vi "Error.Format.vi"(5 "[user-defined descriptions]":string[](array[string]), 7 "[user-defined codes]":i32[](array[numeric]), 8 "error in (no error)":errorcluster, 10 "[error source] (\" \")":string, 11 "[error code] (0)":i32 format="%0.0f") -> (0 "error out":errorcluster, 1 "source out":string, 2 "code out":i32 format="%0.0f", 3 "error?":bool, 4 "message":string=" INSTRUCTIONS:\r\rNormal Use:  When using subVIs that incorporate the error in/error out (or error I/O) structure, place this handler where you want to inform the user of an error, typically at the end of the I/O data path, as the last action of the program.  If the error in error? is ERROR, the handler creates a message describing the error and its source.  If the type of dialog = 1 (default), the message is displayed to the user, who can only acknowedge it.  If the type = 2, the user can acknowledge the message or abort execution; aborting a program with active I/O is not recommended.  If the type = 0, no message is displayed; this is used to process the error programmatically, and the error out cluster elements are wired to individual terminals for that reason.  \r\rOther Use:\n\r\nlocal testing.  To test the error code of a subVI or function that does not have the error I/O structure, you can wire its error code and a source string to the local error code and error source inputs.  If error in error? indicates no error and error code is not equal to 0, the local code and source are substituted for the error in values, and error? is set TRUE (ERROR).")   [LabVIEW 2023, in "VS Plugin Inline Async API.lvlib"]
uses:
  VS Plugin Inline Async API.lvlib
  <vilib>/Utility/error.llb/whitespace.ctl
  <vilib>/Utility/error.llb/Trim Whitespace One-Sided.vi
  <vilib>/Utility/error.llb/Find Tag.vi
panel:
  in  "prompts":T1={"Error %d occurred at %s"="Error %d occurred at %s", "Warning %d occurred at %s"="Warning %d occurred at %s", "Possible reasons: %s"="<b>Possible reason(s):</b>\\n%s", "Error not listed"="This error code is undefined. Undefined errors might occur for a number of reasons. For example, no one has provided a description for the code, or you might have wired a number that is not an error code to the error code input. \n\nAdditionally, undefined error codes might occur because the error relates to a third-party object, such as the operating system or ActiveX. For these third-party errors, you might be able to obtain a description of the error by searching the Web for the error code (%s) or for its hexadecimal representation (0x%s).", "GetCommError x%lx"="Windows GetCommError:  The hex value of this code is <B>x%04lx</B>.\n\nInterpret it bit-wise as follows:\n<B>x4000</B>: serial port VI error\n<B>x0001</B>: receiving queue overflowed or character was received after end-of-file character\n<B>x0002</B>: character was lost by overwrite\n<B>x0004</B>: parity error\n<B>x0008</B>: framing error\n<B>x0010</B>: break condition\n<B>x0020</B>: CTS timeout\n<B>x0040</B>: DSR timeout\n<B>x0080</B>: RLSD timeout\n<B>x0100</B>: transmission queue was full when new character arrived\n<B>x0200</B>: parallel device timeout\n<B>x0400</B>: parallel device I/O error\n<B>x0800</B>: parallel device not selected\n<B>x1000</B>: parallel device out of paper\n<B>x8000</B>: requested mode is  not supported or the idComDev parameter is invalid.", "Continue"="Continue", "Stop"="Stop", "an unidentified location"="an unidentified location", "No Error"="No Error", "Help"="Why not found?"}
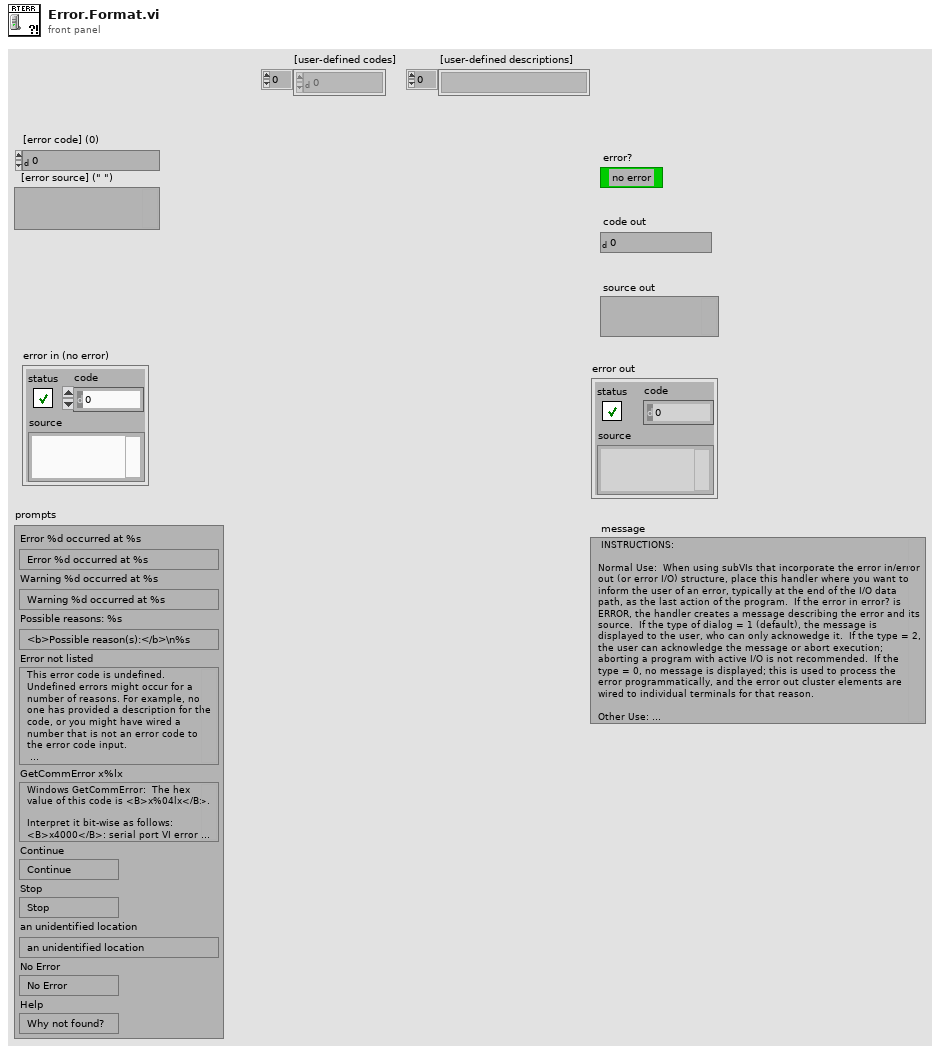
[diagram p1: front panel]
types:
  T1 = cluster{"Error %d occurred at %s":string, "Warning %d occurred at %s":string, "Possible reasons: %s":string, "Error not listed":string, "GetCommError x%lx":string, "Continue":string, "Stop":string, "an unidentified location":string, "No Error":string, "Help":string}
  T2 = typedef "whitespace.ctl" = u16
  T3 = typedef "TagReturnType.ctl" = enum16{"No Tag", "<err>", "<append>"}
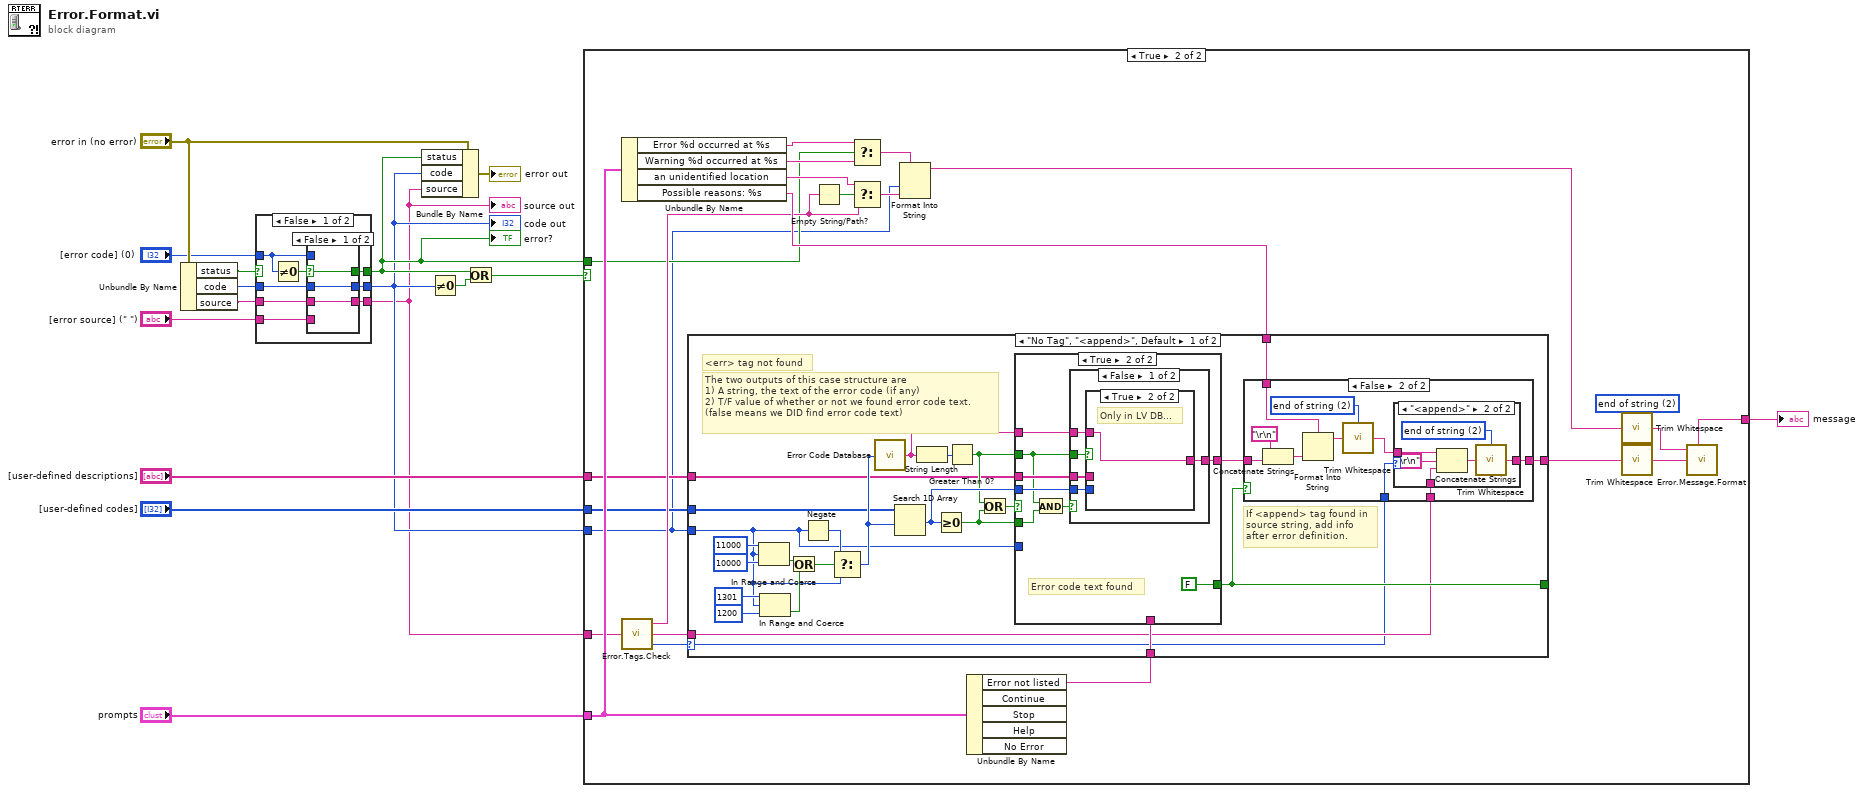
[diagram p0: block diagram]
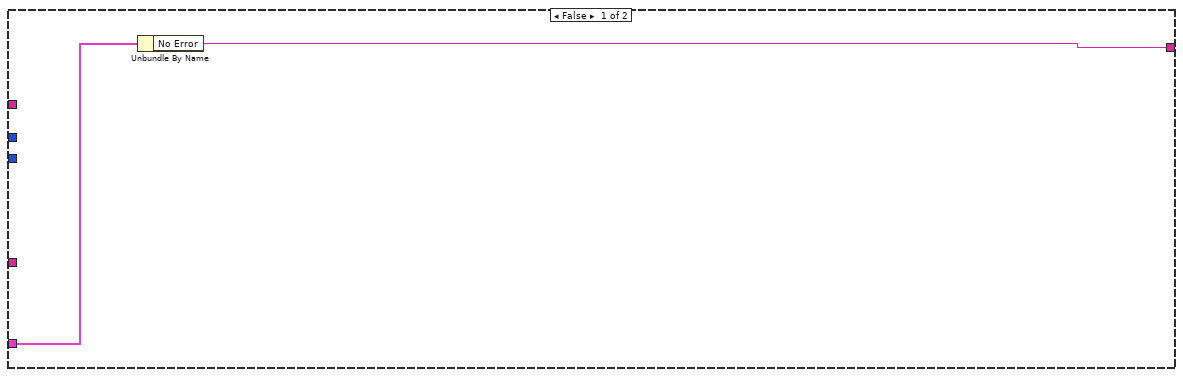
[diagram p4: hidden frame]
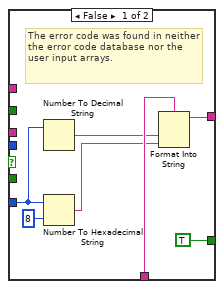
[diagram p7: hidden frame]
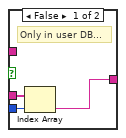
[diagram p8: hidden frame]
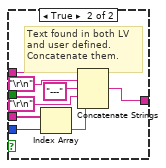
[diagram p9: hidden frame]
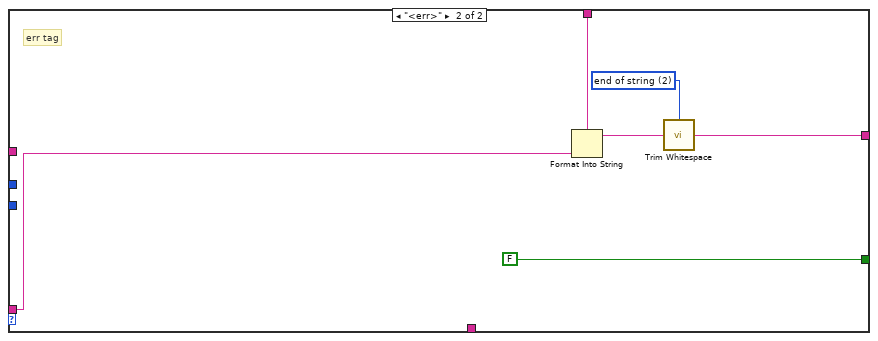
[diagram p10: hidden frame]
diagram:
  n1 = Unbundle By Name("error in (no error)") -> ("status"=w12:bool, "code"=w15:i32, "source"=w16:string)
  n2 = case shown="False" w12 {
    selector: w12 -> [_ w33]
    tunnel: [w22 w32] -> w2
    tunnel: [w23 w33] -> w3
    tunnel: w15 -> [w19 w32]
    tunnel: [w21 w31] -> w1
    tunnel: w16 -> [w20 w31]
    tunnel: "[error code] (0)" -> [w18 _]
    tunnel: "[error source] (\" \")" -> [w17 _]
    frame False {
      n3 = Not Equal To 0?(x=w18) -> (x != 0?=w24:bool)
      n4 = case shown="False" w24 {
        selector: w24 -> [w27 w30]
        tunnel: [w27 w30] -> w23
        tunnel: w18 -> [_ w29]
        tunnel: [w25 w29] -> w22
        tunnel: w17 -> [_ w28]
        tunnel: [w26 w28] -> w21
        tunnel: w20 -> [w26 _]
        tunnel: w19 -> [w25 _]
        frame False {
        }
        frame True {
        }
      }
    }
    frame True {
    }
  }
  "source out" <- w1
  "error?" <- w3
  "code out" <- w2
  n5 = Bundle By Name(cluster="error in (no error)", "status"=w3, "code"=w2, "source"=w1) -> (→"error out":errorcluster)
  n6 = Not Equal To 0?(x=w2) -> (x != 0?=w9:bool)
  n7 = Or(x=w3, y=w9) -> (x .or. y?=w14:bool)
  n8 = case shown="True" w14 {
    tunnel: [w34 w49] -> w5
    tunnel: w3 -> [_ w41]
    tunnel: w1 -> [_ w46]
    tunnel: "prompts" -> [w35 w51]
    tunnel: w2 -> [_ w40]
    tunnel: "[user-defined descriptions]" -> [_ w43]
    tunnel: "[user-defined codes]" -> [_ w42]
    frame False {
      n9 = Unbundle By Name(w35) -> ("No Error"=w34:string)
    }
    frame True {
      w36 = T2 2 items=["both", "start of string", "end of string"] ("location (both)")
      n10 = Unbundle By Name(w51) -> ("Error %d occurred at %s"=w44:string, "Warning %d occurred at %s"=w56:string, "an unidentified location"=w53:string, "Possible reasons: %s"=w50:string)
      n11 = call "Error.Tags.Check.vi"("source"=w46) -> ("Before Tag (source)"=w45:string, "After Tag (special data)"=w57:string, "Tag Found?"=w39:T3)
      n12 = Empty String/Path?(string/path=w45) -> (empty?=w58:bool)
      n13 = Select(t=w44, s=w41, f=w56) -> (s? t:f=w55:string)
      n14 = Select(t=w53, s=w58, f=w45) -> (s? t:f=w54:string)
      n15 = Format Into String(format string=w55, w40, w54) -> (resulting string=w47:string)  [unwired: 2 in, 1 out]
      n16 = Unbundle By Name(w51) -> ("Error not listed"=w52:string)  [unwired: 4 out]
      n17 = case shown="\"No Tag\", \"<append>\", Default" w39 {
        selector: w39 -> [w59 _]
        tunnel: [w64 w137] -> w48
        tunnel: w40 -> [w60 _]
        tunnel: w57 -> [w65 w136]
        tunnel: w52 -> [w83 _]
        tunnel: [w66 FALSE] -> _
        tunnel: w50 -> [w68 w135]
        tunnel: w43 -> [w62 _]
        tunnel: w42 -> [w61 _]
        frame "No Tag", "<append>", Default {
          # "If <append> tag found in source string, add info after error definition."
          # "<err> tag not found"
          # "The two outputs of this case structure are\n1) A string, the text of the error code (if any)\n2) T/F value of whether or not we found error code text.\n(false means we DID find error code text)"
          n18 = In Range and Coerce(upper limit=11000, x=w60, lower limit=10000) -> (In Range?=w76:bool)  [unwired: 1 out]
          n19 = In Range and Coerce(upper limit=1301, x=w60, lower limit=1200) -> (In Range?=w77:bool)  [unwired: 1 out]
          n20 = Or(x=w76, y=w77) -> (x .or. y?=w75:bool)
          n21 = Negate(x=w60) -> (-x=w79:i32)
          n22 = Select(t=w79, s=w75, f=w60) -> (s? t:f=w63:i32)
          n23 = call <vilib>:"Error Code Database.vi"("Error Code"=w63) -> ("Error Text"=w69:string)
          n24 = Search 1D Array(1D array=w61, element=w63) -> (index of element=w82:i32)  [unwired: 1 in]
          n25 = String Length(string=w69) -> (length=w73:i32)
          n26 = Greater Or Equal To 0?(x=w82) -> (x >= 0?=w70:bool)
          n27 = Greater Than 0?(x=w73) -> (x > 0?=w71:bool)
          n28 = Or(x=w71, y=w70) -> (x .or. y?=w72:bool)
          n29 = case shown="True" w72 {
            tunnel: w82 -> [_ w112]
            tunnel: [w106 w110] -> w67
            tunnel: w83 -> [w105 _]
            tunnel: [TRUE FALSE] -> w66
            tunnel: w71 -> [_ w109]
            tunnel: w70 -> [_ w114]
            tunnel: w62 -> [_ w113]
            tunnel: w69 -> [_ w111]
            tunnel: w60 -> [w102 _]
            frame False {
              # "The error code was found in neither the error code database nor the user input arrays."
              n30 = Number To Decimal String(number=w102) -> (decimal integer string=w103:string)  [unwired: 1 in]
              n31 = Number To Hexadecimal String(1:i16 8 ("width (-)"), 2:w102) -> (0:w104:string)
              n32 = Format Into String(format string=w105, w103, w104) -> (resulting string=w106:string)  [unwired: 2 in, 1 out]
            }
            frame True {
              # "Error code text found"
              n33 = And(x=w109, y=w114) -> (x .and. y?=w115:bool)
              n34 = case shown="False" w115 {
                tunnel: w113 -> [w118 w133]
                tunnel: w112 -> [w117 w132]
                tunnel: w111 -> [w119 w126]
                tunnel: [w120 w130] -> w110
                tunnel: w109 -> [w121 _]
                frame False {
                  n35 = case shown="True" w121 {
                    tunnel: [w122 w125] -> w120
                    tunnel: w119 -> [_ w125]
                    tunnel: w118 -> [w124 _]
                    tunnel: w117 -> [w123 _]
                    frame False {
                      # "Only in user DB..."
                      n36 = Index Array(array=w124, index=w123) -> (element=w122:string)
                    }
                    frame True {
                      # "Only in LV DB..."
                    }
                  }
                }
                frame True {
                  # "Text found in both LV\nand user defined. \nConcatenate them."
                  n37 = Index Array(array=w133, index=w132) -> (element=w131:string)
                  n38 = Concatenate Strings(w126, "\r\n" ("End of Line Constant"), "---" ("string"), "\r\n" ("End of Line Constant"), w131) -> (w130:string)
                }
              }
            }
          }
          n39 = case shown="False" w66 {
            tunnel: w68 -> [_ w94]
            tunnel: [w84 w86] -> w64
            tunnel: w67 -> [w84 w91]
            tunnel: w59 -> [_ w88]
            tunnel: w65 -> [_ w87]
            frame True {
              # "no explanation given for error."
            }
            frame False {
              w85 = T2 2 items=["both", "start of string", "end of string"] ("location (both)")
              n40 = Concatenate Strings("\r\n" ("End of Line Constant"), w91) -> (w92:string)
              n41 = Format Into String(format string=w94, w92) -> (resulting string=w93:string)  [unwired: 2 in, 1 out]
              n42 = call <vilib>:"Trim Whitespace.vi"("string"=w93, "location (both)"=w85) -> ("trimmed string"=w89:string)
              n43 = case shown="\"<append>\"" w88 {
                tunnel: w89 -> [w95 w100]
                tunnel: [w95 w97] -> w86
                tunnel: w87 -> [_ w99]
                frame "No Tag", Default {
                }
                frame "<append>" {
                  w96 = T2 2 items=["both", "start of string", "end of string"] ("location (both)")
                  n44 = Concatenate Strings(w100, "\r\n" ("End of Line Constant"), w99) -> (w98:string)
                  n45 = call <vilib>:"Trim Whitespace.vi"("string"=w98, "location (both)"=w96) -> ("trimmed string"=w97:string)
                }
              }
            }
          }
        }
        frame "<err>" {
          w134 = T2 2 items=["both", "start of string", "end of string"] ("location (both)")
          # "err tag"
          n46 = Format Into String(format string=w135, w136) -> (resulting string=w138:string)  [unwired: 2 in, 1 out]
          n47 = call <vilib>:"Trim Whitespace.vi"("string"=w138, "location (both)"=w134) -> ("trimmed string"=w137:string)
        }
      }
      n48 = call <vilib>:"Trim Whitespace.vi"("string"=w47, "location (both)"=w36) -> ("trimmed string"=w37:string)
      n49 = call <vilib>:"Trim Whitespace.vi"("string"=w48, "location (both)"=w36) -> ("trimmed string"=w38:string)
      n50 = call "Error.Message.Format.vi"("Source"=w37, "Details"=w38) -> ("message"=w49:string)  [unwired: 2 in, 4 out]
    }
  }
  "message" <- w5
